vi "nanocal_process tdms folder.vi"() -> ()   [LabVIEW 2021]
uses:
  NHMFL_Core/Libraries/File/File Format Converter/Format Converter Configuration.ctl
  nanocal_process_tdms_file_control.ctl
panel:
  out "current file index":i32
  out "current file":path
  out "# of files":i32
  out "All Files in Dir":path[](array[path])
  out "ALL channel names":string[](array[string])
  out "new Configuration":T1={"New start time"=nan, "New end time"=nan, "Output file format"=enum."ASCII", "Save ASCII column names"=TRUE, "Prepend binary array size"=FALSE, "buffer size (-1: all)"=100000, "Group"="p", "New dt"=nan, "IGORify column names"=TRUE, "eliminate spaces in col name"=TRUE, "Channels"=[]} {"buffer size (-1: all)" format="%.0p"; "New start time" format="%#_10p"}
  in  "pattern":string="m*_*.tdms"
  in  "Configuration":T1={"New start time"=nan, "New end time"=nan, "Output file format"=enum."ASCII", "Save ASCII column names"=TRUE, "Prepend binary array size"=FALSE, "buffer size (-1: all)"=100000, "Group"="p", "New dt"=nan, "IGORify column names"=TRUE, "eliminate spaces in col name"=TRUE, "Channels"=["jsdhgv", "lsjdfh", "ajlsd"]} {"buffer size (-1: all)" format="%.0p"; "New start time" format="%#_10p"}
  in  "Folder Path":path=path "/Users/arkadyshekhter/Library/CloudStorage/Dropbox/shared_Ali/nanocal-March2020 - RuCl3/March_2020"
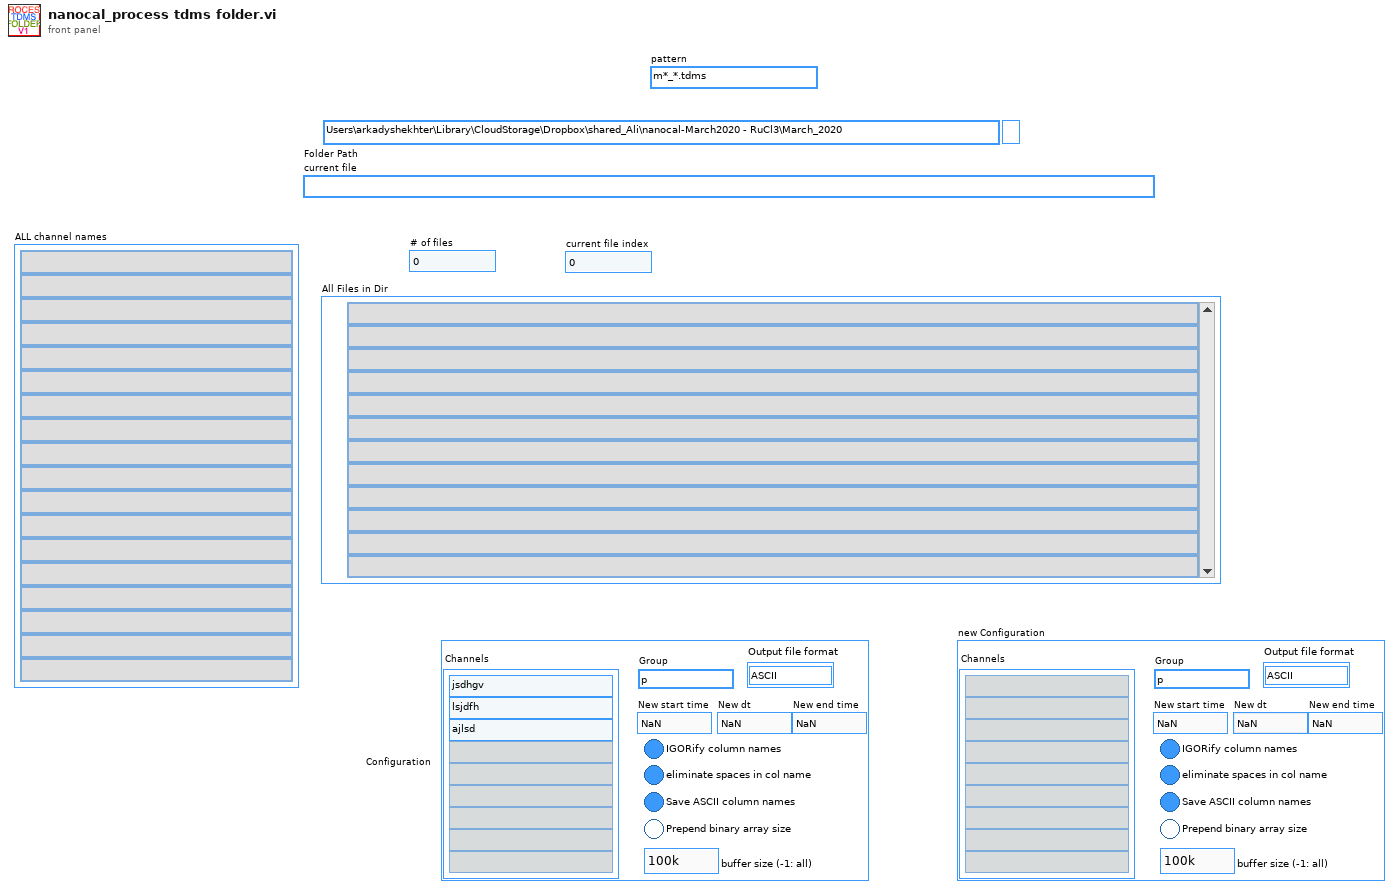
[diagram p1: front panel]
types:
  T1 = typedef "Format Converter Configuration.ctl" = cluster{"New start time":dbl, "New end time":dbl, "Output file format":enum16{"ASCII", "BINARY", "TDMS"}, "Save ASCII column names":bool, "Prepend binary array size":bool, "buffer size (-1: all)":i64, "Group":string, "New dt":dbl, "IGORify column names":bool, "eliminate spaces in col name":bool, "Channels":string[]}
  T2 = typedef "nanocal_process_tdms_file_control.ctl" = enum16{"all fileds", "subset of fields"}
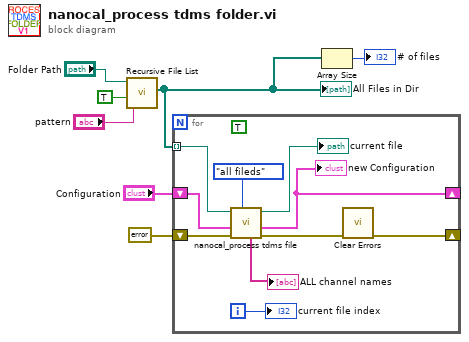
[diagram p0: block diagram]
diagram:
  n1 = call <vilib>:"Recursive File List.vi"("pattern"="pattern", "Continue Recursing on Error? (F)"=TRUE, "Folder Path"="Folder Path") -> ("All Files in Dir"=w1:path[])  [unwired: 4 in, 4 out]
  "All Files in Dir" <- w1
  n2 = for {
    tunnel: w1 -> [w15] mode=indexing
    shift-right: [w17] -> _
    shift-left: errorcluster {"status"=FALSE, "code"=0, "source"=""} ("Error In") -> [w14]
    shift-right: [w10] -> _
    shift-left: "Configuration" -> [w12]
    i -> [w16]
    (unwired) TRUE
    n3 = call "nanocal_process tdms file.vi"("actions"=nanocal_process_tdms_file_control."all fileds", "Error In"=w14, "Configuration"=w12, "tdms file IN"=w15) -> ("Error Out"=w11:errorcluster, "new Configuration"=w10:T1, "tdms file OUT"=→"current file":path, "ALL channel names"=→"ALL channel names":string[])  [unwired: 3 in, 1 out]
    "new Configuration" <- w10
    n4 = call <vilib>:"Clear Errors.vi"("error in (no error)"=w11) -> ("error out"=w17:errorcluster)  [unwired: 5 in, 1 out]
    "current file index" <- w16
  }
  n5 = Array Size(array=w1) -> (size(s)=→"# of files":i32)
